vi "叶绿素a_获取温度和叶绿素值.vi"(8 "error in (no error)":errorcluster caption="错误输入（无错误）", 11 "MB session in":refnum<class "MB_Master.lvclass">) -> (0 "error out":errorcluster caption="错误输出", 2 "输出值":cluster{"温度测量值":sgl, "叶绿素测量值":sgl, "错误标志":u16} {"错误标志" items=["NO Error"=0, "刷子没到位"=255]}, 3 "MB session out":refnum<class "MB_Master.lvclass">)   [LabVIEW 2016, in "斯坦道多参数.lvlib"]
uses:
  <vilib>/Plasmionique/MB Master/MB_Master/MB_Master.lvclass
  <vilib>/Plasmionique/MB Master/MB Master.lvlib
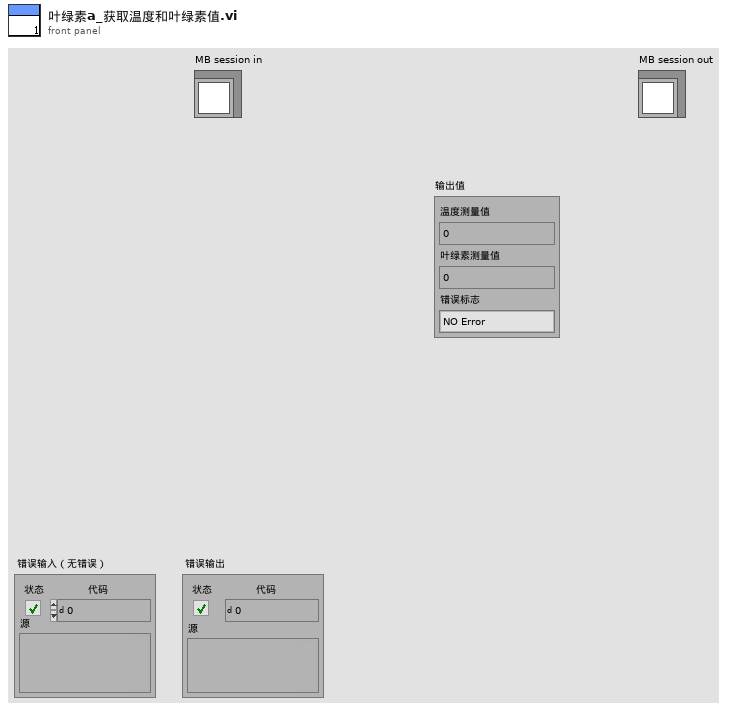
[diagram p1: front panel]
types:
  T1 = cluster{"pH":u32, "DO":u32, "Cond":u32, "Turb":u32, "叶绿素a":u32, "藻密度":u32, "ORP":u32, "COD":u32}
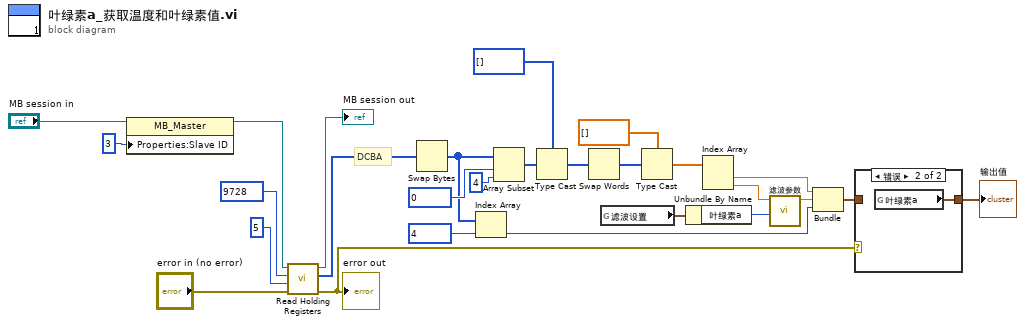
[diagram p0: block diagram]
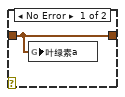
[diagram p2: hidden frame]
diagram:
  # "DCBA"
  n1 = property class="MB_Master"(reference="MB session in", "Properties:Slave ID"=u16 3 ("y")) -> (reference out=w16:refnum<class "MB_Master.lvclass">)  [unwired: 1 in, 1 out]
  n2 = call <vilib>:"Read Holding Registers.vi"("error in (no error)"="error in (no error)", "quantity"=u16 5, "starting address"=u16 9728, "MB session in"=w16) -> ("error out"=w9:errorcluster, "Registers"=w12:u16[], "MB session out"=→"MB session out":refnum<class "MB_Master.lvclass">)  [unwired: 5 in]
  "error out" <- w9
  n3 = Swap Bytes(anything=w12) -> (byte swapped=w11:u16[])
  n4 = Index Array(array=w11, index=u16 4 ("starting address")) -> (element=w13:u16)
  n5 = Array Subset(array=w11, index=u16 0 ("starting address"), length=4 ("长度")) -> (w10:u16[])
  n6 = Type Cast(type=u32[] [] ("数组 2"), x=w10) -> (*(type *) &x=w22:u32[])
  n7 = Swap Words(1:w22) -> (0:w24:u32[])
  n8 = global read "断电保存变量.vi" "滤波设置"() -> (w3:T1)
  n9 = Type Cast(type=sgl[] [] ("数组 2"), x=w24) -> (*(type *) &x=w20:sgl[])
  n10 = Unbundle By Name(w3) -> ("叶绿素a"=w2:u32)
  n11 = Index Array(array=w20) -> (element #1=w19:sgl, element #2=w5:sgl)  [unwired: 2 in]
  n12 = call "滤波参数.vi"("滤波次数"=w2, "x"=w5) -> ("mode"=w4:dbl)  [unwired: 9 in]
  n13 = Bundle("数值"=w19, "mode"=w4, w13) -> (w8:cluster{"数值":sgl, "mode":dbl, u16})  [unwired: 1 in]
  n14 = case shown="错误" w9 {
    tunnel: w8 -> [w28 _]
    tunnel: [w28 w29] -> w1
    frame No Error {
      n15 = global write "禹山过程全局变量.vi" "叶绿素a"(w28) -> ()
    }
    frame Error {
      n16 = global read "禹山过程全局变量.vi" "叶绿素a"() -> (w29:cluster{"温度测量值":sgl, "叶绿素测量值":sgl, "错误标志":u16})
    }
  }
  "输出值" <- w1
